vi "slscsl_relayControl.vi"(8 "error in (no error)":errorcluster, 9 "relay action (Close Relay)":T1=enum."Close Relay", 10 "relayNames":string, 11 "Route Manager in":refnum<class "slscsl.lvclass">) -> (0 "error out":errorcluster, 3 "Route Manager out":refnum<class "slscsl.lvclass">)   [LabVIEW 2015, in "slscsl.lvclass"]
uses:
  slscsl.lvclass
  RelayAction.ctl
  slscsl.lvclass/slscsl.ctl
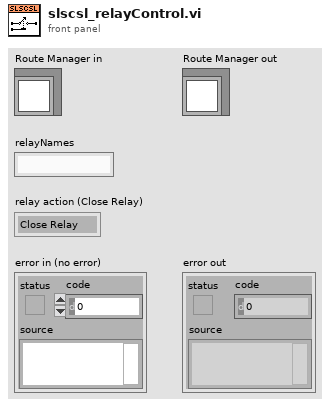
[diagram p1: front panel]
types:
  T1 = typedef "slscsl.lvclass/RelayAction.ctl" = enum16{"Open Relay", "Close Relay"}
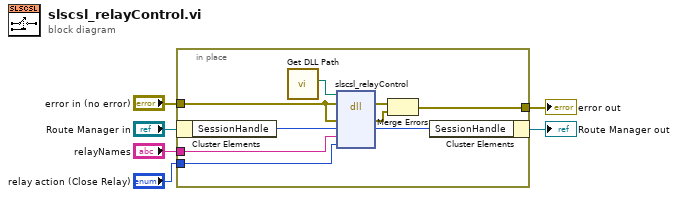
[diagram p0: block diagram]
diagram:
  n1 = in-place {
    in-place-border: "error in (no error)" -> [w12]
    in-place-border: [w11] -> w5
    in-place-border: "relayNames" -> [w8]
    in-place-border: "relay action (Close Relay)" -> [w7]
    n2 = in-place-cluster #1("Route Manager in") -> ("SessionHandle"=w10:u64)
    n3 = call "Get DLL Path.vi"() -> ("slscsl DLL Path"=w13:path)  [unwired: 11 in]
    n4 = dll-call lib="?" fn="slscsl_relayControl"(path in=w13, error in=w12, "errorCluster"=w12, "sessionHandle"=w10, "relayNames"=w8, "relayActions"=w7) -> (error out=w15:errorcluster, "errorCluster"=w14:errorcluster, "sessionHandle"=w9:u64)  [unwired: 4 in, 1 out]
    n5 = Merge Errors(w15, w14) -> (w11:errorcluster)
    n6 = in-place-cluster #1("SessionHandle"=w9) -> (→"Route Manager out":refnum<class "slscsl.lvclass">)
  }
  "error out" <- w5
